vi "GeoData.vi"() -> ()   [LabVIEW 2017] (continued)
FL\tOrange County\tH1\n32733\t12095\tGoldenrod\tFL\tOrange County\tH1\n32792\t12095\tWinter park\tFL\tOrange County\tH1\n32768\t12095\tPlymouth\tFL\tOrange County\tH1\n32794\t12095\tMaitland\tFL\tOrange County\tH1\n32704\t12095\tApopka\tFL\tOrange County\tH1\n32709\t12095\tChristmas\tFL\tOrange County\tH1\n32818\t12095\tOrlando\tFL\tOrange County\tH1\n32803\t12095\tOrlando\tFL\tOrange County\tH1\n32806\t12095\tOrlando\tFL\tOrange County\tH1\n34761\t12095\tOcoee\tFL\tOrange County\tH1\n34786\t12095\tWindermere\tFL\tOrange County\tH1\n32856\t12095\tOrlando\tFL\tOrange County\tH1\n32703\t12095\tApopka\tFL\tOrange County\tH1\n32814\t12095\tOrlando\tFL\tOrange County\tH1\n32805\t12095\tOrlando\tFL\tOrange County\tH1\n32821\t12095\tOrlando\tFL\tOrange County\tH1\n32822\t12095\tOrlando\tFL\tOrange County\tH1\n32826\t12095\tOrlando\tFL\tOrange County\tH1\n32837\t12095\tOrlando\tFL\tOrange County\tH1\n32868\t12095\tOrlando\tFL\tOrange County\tH1\n32872\t12095\tOrlando\tFL\tOrange County\tH1\n32751\t12095\tMaitland\tFL\tOrange County\tH1\n32757\t12095\tMount dora\tFL\tOrange County\tH1\n34734\t12095\tGotha\tFL\tOrange County\tH1\n32860\t12095\tOrlando\tFL\tOrange County\tH1\n32802\t12095\tOrlando\tFL\tOrange County\tH1\n34778\t12095\tWinter garden\tFL\tOrange County\tH1\n32790\t12095\tWinter park\tFL\tOrange County\tH1\n34740\t12095\tKillarney\tFL\tOrange County\tH1\n32834\t12095\tOrlando\tFL\tOrange County\tH1\n32812\t12095\tOrlando\tFL\tOrange County\tH1\n32825\t12095\tOrlando\tFL\tOrange County\tH1\n32819\t12095\tOrlando\tFL\tOrange County\tH1\n32810\t12095\tOrlando\tFL\tOrange County\tH1\n32869\t12095\tOrlando\tFL\tOrange County\tH1\n32829\t12095\tOrlando\tFL\tOrange County\tH1\n32857\t12095\tOrlando\tFL\tOrange County\tH1\n32862\t12095\tOrlando\tFL\tOrange County\tH1\n32808\t12095\tOrlando\tFL\tOrange County\tH1\n32809\t12095\tOrlando\tFL\tOrange County\tH1\n32811\t12095\tOrlando\tFL\tOrange County\tH1\n32827\t12095\tOrlando\tFL\tOrange County\tH1\n32807\t12095\tOrlando\tFL\tOrange County\tH1\n32801\t12095\tOrlando\tFL\tOrange County\tH1\n32839\t12095\tOrlando\tFL\tOrange County\tH1\n32853\t12095\tOrlando\tFL\tOrange County\tH1\n32833\t12095\tOrlando\tFL\tOrange County\tH1\n34787\t12095\tWinter garden\tFL\tOrange County\tH1\n32855\t12095\tOrlando\tFL\tOrange County\tH1\n32816\t12095\tOrlando\tFL\tOrange County\tH1\n32878\t12095\tOrlando\tFL\tOrange County\tH1\n32712\t12095\tApopka\tFL\tOrange County\tH1\n32836\t12095\tOrlando\tFL\tOrange County\tH1\n32820\t12095\tOrlando\tFL\tOrange County\tH1\n32789\t12095\tWinter park\tFL\tOrange County\tH1\n32859\t12095\tOrlando\tFL\tOrange County\tH1\n32854\t12095\tOrlando\tFL\tOrange County\tH1\n32831\t12095\tOrlando\tFL\tOrange County\tH1\n34746\t12097\tKissimmee\tFL\tOsceola County\tH1\n34747\t12097\tKissimmee\tFL\tOsceola County\tH1\n34742\t12097\tKissimmee\tFL\tOsceola County\tH1\n34745\t12097\tKissimmee\tFL\tOsceola County\tH1\n32830\t12097\tOrlando\tFL\tOsceola County\tH1\n34972\t12097\tOkeechobee\tFL\tOsceola County\tH1\n34741\t12097\tKissimmee\tFL\tOsceola County\tH1\n34769\t12097\tSaint cloud\tFL\tOsceola County\tH1\n34771\t12097\tSaint cloud\tFL\tOsceola County\tH1\n34744\t12097\tKissimmee\tFL\tOsceola County\tH1\n33848\t12097\tIntercession city\tFL\tOsceola County\tH1\n32821\t12097\tOrlando\tFL\tOsceola County\tH1\n32837\t12097\tOrlando\tFL\tOsceola County\tH1\n34714\t12097\tClermont\tFL\tOsceola County\tH1\n33897\t12097\tDavenport\tFL\tOsceola County\tH1\n34739\t12097\tKenansville\tFL\tOsceola County\tH1\n34773\t12097\tSaint cloud\tFL\tOsceola County\tH1\n34743\t12097\tKissimmee\tFL\tOsceola County\tH1\n34759\t12097\tKissimmee\tFL\tOsceola County\tH1\n34758\t12097\tKissimmee\tFL\tOsceola County\tH1\n34772\t12097\tSaint cloud\tFL\tOsceola County\tH1\n34770\t12097\tSaint cloud\tFL\tOsceola County\tH1\n33896\t12097\tDavenport\tFL\tOsceola County\tH1\n33403\t12099\tWest palm beach\tFL\tPalm Beach County\tH1\n33409\t12099\tWest palm beach\tFL\tPalm Beach County\tH1\n33412\t12099\tWest palm beach\tFL\tPalm Beach County\tH1\n33415\t12099\tWest palm beach\tFL\tPalm Beach County\tH1\n33417\t12099\tWest palm beach\tFL\tPalm Beach County\tH1\n33446\t12099\tDelray beach\tFL\tPalm Beach County\tH1\n33460\t12099\tLake worth\tFL\tPalm Beach County\tH1\n33434\t12099\tBoca raton\tFL\tPalm Beach County\tH1\n33436\t12099\tBoynton beach\tFL\tPalm Beach County\tH1\n33478\t12099\tJupiter\tFL\tPalm Beach County\tH1\n33476\t12099\tPahokee\tFL\tPalm Beach County\tH1\n33484\t12099\tDelray beach\tFL\tPalm Beach County\tH1\n33488\t12099\tBoca raton\tFL\tPalm Beach County\tH1\n33448\t12099\tDelray beach\tFL\tPalm Beach County\tH1\n33401\t12099\tWest palm beach\tFL\tPalm Beach County\tH1\n33411\t12099\tWest palm beach\tFL\tPalm Beach County\tH1\n33425\t12099\tBoynton beach\tFL\tPalm Beach County\tH1\n33435\t12099\tBoynton beach\tFL\tPalm Beach County\tH1\n33444\t12099\tDelray beach\tFL\tPalm Beach County\tH1\n33449\t12099\tLake worth\tFL\tPalm Beach County\tH1\n33487\t12099\tBoca raton\tFL\tPalm Beach County\tH1\n33464\t12099\tBoca raton\tFL\tPalm Beach County\tH1\n33413\t12099\tWest palm beach\tFL\tPalm Beach County\tH1\n33429\t12099\tBoca raton\tFL\tPalm Beach County\tH1\n33472\t12099\tBoynton beach\tFL\tPalm Beach County\tH1\n33498\t12099\tBoca raton\tFL\tPalm Beach County\tH1\n33497\t12099\tBoca raton\tFL\tPalm Beach County\tH1\n33410\t12099\tPalm beach gardens\tFL\tPalm Beach County\tH1\n33427\t12099\tBoca raton\tFL\tPalm Beach County\tH1\n33445\t12099\tDelray beach\tFL\tPalm Beach County\tH1\n33463\t12099\tLake worth\tFL\tPalm Beach County\tH1\n33473\t12099\tBoynton beach\tFL\tPalm Beach County\tH1\n33480\t12099\tPalm beach\tFL\tPalm Beach County\tH1\n33465\t12099\tLake worth\tFL\tPalm Beach County\tH1\n33499\t12099\tBoca raton\tFL\tPalm Beach County\tH1\n33405\t12099\tWest palm beach\tFL\tPalm Beach County\tH1\n33414\t12099\tWellington\tFL\tPalm Beach County\tH1\n33431\t12099\tBoca raton\tFL\tPalm Beach County\tH1\n33462\t12099\tLake worth\tFL\tPalm Beach County\tH1\n33467\t12099\tLake worth\tFL\tPalm Beach County\tH1\n33438\t12099\tCanal point\tFL\tPalm Beach County\tH1\n33486\t12099\tBoca raton\tFL\tPalm Beach County\tH1\n33493\t12099\tSouth bay\tFL\tPalm Beach County\tH1\n33468\t12099\tJupiter\tFL\tPalm Beach County\tH1\n33418\t12099\tPalm beach gardens\tFL\tPalm Beach County\tH1\n33430\t12099\tBelle glade\tFL\tPalm Beach County\tH1\n33440\t12099\tClewiston\tFL\tPalm Beach County\tH1\n33458\t12099\tJupiter\tFL\tPalm Beach County\tH1\n33461\t12099\tLake worth\tFL\tPalm Beach County\tH1\n33433\t12099\tBoca raton\tFL\tPalm Beach County\tH1\n33477\t12099\tJupiter\tFL\tPalm Beach County\tH1\n33496\t12099\tBoca raton\tFL\tPalm Beach County\tH1\n33466\t12099\tLake worth\tFL\tPalm Beach County\tH1\n33454\t12099\tGreenacres\tFL\tPalm Beach County\tH1\n33407\t12099\tWest palm beach\tFL\tPalm Beach County\tH1\n33421\t12099\tRoyal palm beach\tFL\tPalm Beach County\tH1\n33406\t12099\tWest palm beach\tFL\tPalm Beach County\tH1\n33419\t12099\tWest palm beach\tFL\tPalm Beach County\tH1\n33437\t12099\tBoynton beach\tFL\tPalm Beach County\tH1\n33482\t12099\tDelray beach\tFL\tPalm Beach County\tH1\n33404\t12099\tWest palm beach\tFL\tPalm Beach County\tH1\n33408\t12099\tNorth palm beach\tFL\tPalm Beach County\tH1\n33428\t12099\tBoca raton\tFL\tPalm Beach County\tH1\n33426\t12099\tBoynton beach\tFL\tPalm Beach County\tH1\n33402\t12099\tWest palm beach\tFL\tPalm Beach County\tH1\n33416\t12099\tWest palm beach\tFL\tPalm Beach County\tH1\n33424\t12099\tBoynton beach\tFL\tPalm Beach County\tH1\n33432\t12099\tBoca raton\tFL\tPalm Beach County\tH1\n33469\t12099\tJupiter\tFL\tPalm Beach County\tH1\n33470\t12099\tLoxahatchee\tFL\tPalm Beach County\tH1\n33483\t12099\tDelray beach\tFL\tPalm Beach County\tH1\n33481\t12099\tBoca raton\tFL\tPalm Beach County\tH1\n33422\t12099\tWest palm beach\tFL\tPalm Beach County\tH1\n33474\t12099\tBoynton beach\tFL\tPalm Beach County\tH1\n33420\t12099\tWest palm beach\tFL\tPalm Beach County\tH1\n33459\t12099\tLake harbor\tFL\tPalm Beach County\tH1\n34653\t12101\tNew port richey\tFL\tPasco County\tH1\n34667\t12101\tHudson\tFL\tPasco County\tH1\n34637\t12101\tLand o lakes\tFL\tPasco County\tH1\n34690\t12101\tHoliday\tFL\tPasco County\tH1\n33523\t12101\tDade city\tFL\tPasco County\tH1\n33597\t12101\tWebster\tFL\tPasco County\tH1\n33544\t12101\tWesley chapel\tFL\tPasco County\tH1\n33548\t12101\tLutz\tFL\tPasco County\tH1\n33524\t12101\tCrystal springs\tFL\tPasco County\tH1\n33593\t12101\tTrilby\tFL\tPasco County\tH1\n33537\t12101\tLacoochee\tFL\tPasco County\tH1\n33558\t12101\tLutz\tFL\tPasco County\tH1\n33525\t12101\tDade city\tFL\tPasco County\tH1\n34610\t12101\tSpring hill\tFL\tPasco County\tH1\n34689\t12101\tTarpon springs\tFL\tPasco County\tH1\n34656\t12101\tNew port richey\tFL\tPasco County\tH1\n33849\t12101\tKathleen\tFL\tPasco County\tH1\n34679\t12101\tAripeka\tFL\tPasco County\tH1\n33545\t12101\tWesley chapel\tFL\tPasco County\tH1\n33539\t12101\tZephyrhills\tFL\tPasco County\tH1\n33526\t12101\tDade city\tFL\tPasco County\tH1\n34692\t12101\tHoliday\tFL\tPasco County\tH1\n33549\t12101\tLutz\tFL\tPasco County\tH1\n33576\t12101\tSan antonio\tFL\tPasco County\tH1\n34652\t12101\tNew port richey\tFL\tPasco County\tH1\n34668\t12101\tPort richey\tFL\tPasco County\tH1\n34674\t12101\tHudson\tFL\tPasco County\tH1\n34673\t12101\tPort richey\tFL\tPasco County\tH1\n33559\t12101\tLutz\tFL\tPasco County\tH1\n33543\t12101\tWesley chapel\tFL\tPasco County\tH1\n33542\t12101\tZephyrhills\tFL\tPasco County\tH1\n34604\t12101\tBrooksville\tFL\tPasco County\tH1\n34654\t12101\tNew port richey\tFL\tPasco County\tH1\n34655\t12101\tNew port richey\tFL\tPasco County\tH1\n34639\t12101\tLand o lakes\tFL\tPasco County\tH1\n34691\t12101\tHoliday\tFL\tPasco County\tH1\n33541\t12101\tZephyrhills\tFL\tPasco County\tH1\n33540\t12101\tZephyrhills\tFL\tPasco County\tH1\n33556\t12101\tOdessa\tFL\tPasco County\tH1\n34638\t12101\tLand o lakes\tFL\tPasco County\tH1\n34669\t12101\tHudson\tFL\tPasco County\tH1\n33809\t12101\tLakeland\tFL\tPasco County\tH1\n34680\t12101\tElfers\tFL\tPasco County\tH1\n33574\t12101\tSaint leo\tFL\tPasco County\tH1\n33701\t12103\tSaint petersburg\tFL\tPinellas County\tH1\n33709\t12103\tSaint petersburg\tFL\tPinellas County\tH1\n33776\t12103\tSeminole\tFL\tPinellas County\tH1\n33763\t12103\tClearwater\tFL\tPinellas County\tH1\n33710\t12103\tSaint petersburg\tFL\tPinellas County\tH1\n33782\t12103\tPinellas park\tFL\tPinellas County\tH1\n33773\t12103\tLargo\tFL\tPinellas County\tH1\n33786\t12103\tBelleair beach\tFL\tPinellas County\tH1\n33734\t12103\tSaint petersburg\tFL\tPinellas County\tH1\n33705\t12103\tSaint petersburg\tFL\tPinellas County\tH1\n33772\t12103\tSeminole\tFL\tPinellas County\tH1\n33713\t12103\tSaint petersburg\tFL\tPinellas County\tH1\n34683\t12103\tPalm harbor\tFL\tPinellas County\tH1\n33742\t12103\tSaint petersburg\tFL\tPinellas County\tH1\n33743\t12103\tSaint petersburg\tFL\tPinellas County\tH1\n33775\t12103\tSeminole\tFL\tPinellas County\tH1\n34682\t12103\tPalm harbor\tFL\tPinellas County\tH1\n33707\t12103\tSaint petersburg\tFL\tPinellas County\tH1\n33733\t12103\tSaint petersburg\tFL\tPinellas County\tH1\n33766\t12103\tClearwater\tFL\tPinellas County\tH1\n33712\t12103\tSaint petersburg\tFL\tPinellas County\tH1\n33747\t12103\tSaint petersburg\tFL\tPinellas County\tH1\n34689\t12103\tTarpon springs\tFL\tPinellas County\tH1\n34697\t12103\tDunedin\tFL\tPinellas County\tH1\n33760\t12103\tClearwater\tFL\tPinellas County\tH1\n34698\t12103\tDunedin\tFL\tPinellas County\tH1\n33738\t12103\tSaint petersburg\tFL\tPinellas County\tH1\n33741\t12103\tSaint petersburg\tFL\tPinellas County\tH1\n33729\t12103\tSaint petersburg\tFL\tPinellas County\tH1\n33730\t12103\tSaint petersburg\tFL\tPinellas County\tH1\n33703\t12103\tSaint petersburg\tFL\tPinellas County\tH1\n33702\t12103\tSaint petersburg\tFL\tPinellas County\tH1\n33715\t12103\tSaint petersburg\tFL\tPinellas County\tH1\n33716\t12103\tSaint petersburg\tFL\tPinellas County\tH1\n33767\t12103\tClearwater beach\tFL\tPinellas County\tH1\n33778\t12103\tLargo\tFL\tPinellas County\tH1\n33781\t12103\tPinellas park\tFL\tPinellas County\tH1\n33744\t12103\tBay pines\tFL\tPinellas County\tH1\n34681\t12103\tCrystal beach\tFL\tPinellas County\tH1\n33626\t12103\tTampa\tFL\tPinellas County\tH1\n33706\t12103\tSaint petersburg\tFL\tPinellas County\tH1\n33755\t12103\tClearwater\tFL\tPinellas County\tH1\n33761\t12103\tClearwater\tFL\tPinellas County\tH1\n33771\t12103\tLargo\tFL\tPinellas County\tH1\n33736\t12103\tSaint petersburg\tFL\tPinellas County\tH1\n33765\t12103\tClearwater\tFL\tPinellas County\tH1\n33756\t12103\tClearwater\tFL\tPinellas County\tH1\n33774\t12103\tLargo\tFL\tPinellas County\tH1\n33785\t12103\tIndian rocks beach\tFL\tPinellas County\tH1\n34677\t12103\tOldsmar\tFL\tPinellas County\tH1\n34685\t12103\tPalm harbor\tFL\tPinellas County\tH1\n34688\t12103\tTarpon springs\tFL\tPinellas County\tH1\n33779\t12103\tLargo\tFL\tPinellas County\tH1\n34660\t12103\tOzona\tFL\tPinellas County\tH1\n33708\t12103\tSaint petersburg\tFL\tPinellas County\tH1\n33757\t12103\tClearwater\tFL\tPinellas County\tH1\n33764\t12103\tClearwater\tFL\tPinellas County\tH1\n33770\t12103\tLargo\tFL\tPinellas County\tH1\n33780\t12103\tPinellas park\tFL\tPinellas County\tH1\n34684\t12103\tPalm harbor\tFL\tPinellas County\tH1\n33758\t12103\tClearwater\tFL\tPinellas County\tH1\n33704\t12103\tSaint petersburg\tFL\tPinellas County\tH1\n33759\t12103\tClearwater\tFL\tPinellas County\tH1\n33711\t12103\tSaint petersburg\tFL\tPinellas County\tH1\n33714\t12103\tSaint petersburg\tFL\tPinellas County\tH1\n33762\t12103\tClearwater\tFL\tPinellas County\tH1\n33777\t12103\tSeminole\tFL\tPinellas County\tH1\n33731\t12103\tSaint petersburg\tFL\tPinellas County\tH1\n34695\t12103\tSafety harbor\tFL\tPinellas County\tH1\n33732\t12103\tSaint petersburg\tFL\tPinellas County\tH1\n33784\t12103\tSaint petersburg\tFL\tPinellas County\tH1\n33547\t12105\tLithia\tFL\tPolk County\tH1\n33843\t12105\tFrostproof\tFL\tPolk County\tH1\n33838\t12105\tDundee\tFL\tPolk County\tH1\n33835\t12105\tBradley\tFL\tPolk County\tH1\n33855\t12105\tIndian lake estates\tFL\tPolk County\tH1\n33844\t12105\tHaines city\tFL\tPolk County\tH1\n33825\t12105\tAvon park\tFL\tPolk County\tH1\n33868\t12105\tPolk city\tFL\tPolk County\tH1\n33804\t12105\tLakeland\tFL\tPolk County\tH1\n33846\t12105\tHighland city\tFL\tPolk County\tH1\n33847\t12105\tHomeland\tFL\tPolk County\tH1\n33854\t12105\tLakeshore\tFL\tPolk County\tH1\n33801\t12105\tLakeland\tFL\tPolk County\tH1\n33837\t12105\tDavenport\tFL\tPolk County\tH1\n33813\t12105\tLakeland\tFL\tPolk County\tH1\n33823\t12105\tAuburndale\tFL\tPolk County\tH1\n33827\t12105\tBabson park\tFL\tPolk County\tH1\n33853\t12105\tLake wales\tFL\tPolk County\tH1\n33841\t12105\tFort meade\tFL\tPolk County\tH1\n33836\t12105\tDavenport\tFL\tPolk County\tH1\n33849\t12105\tKathleen\tFL\tPolk County\tH1\n33820\t12105\tAlturas\tFL\tPolk County\tH1\n33856\t12105\tNalcrest\tFL\tPolk County\tH1\n33863\t12105\tNichols\tFL\tPolk County\tH1\n33805\t12105\tLakeland\tFL\tPolk County\tH1\n33802\t12105\tLakeland\tFL\tPolk County\tH1\n33831\t12105\tBartow\tFL\tPolk County\tH1\n33851\t12105\tLake hamilton\tFL\tPolk County\tH1\n34714\t12105\tClermont\tFL\tPolk County\tH1\n33830\t12105\tBartow\tFL\tPolk County\tH1\n33897\t12105\tDavenport\tFL\tPolk County\tH1\n33812\t12105\tLakeland\tFL\tPolk County\tH1\n33834\t12105\tBowling green\tFL\tPolk County\tH1\n33839\t12105\tEagle lake\tFL\tPolk County\tH1\n33885\t12105\tWinter haven\tFL\tPolk County\tH1\n33840\t12105\tEaton park\tFL\tPolk County\tH1\n33845\t12105\tHaines city\tFL\tPolk County\tH1\n33867\t12105\tRiver ranch\tFL\tPolk County\tH1\n33860\t12105\tMulberry\tFL\tPolk County\tH1\n33810\t12105\tLakeland\tFL\tPolk County\tH1\n33881\t12105\tWinter haven\tFL\tPolk County\tH1\n33898\t12105\tLake wales\tFL\tPolk County\tH1\n33806\t12105\tLakeland\tFL\tPolk County\tH1\n33803\t12105\tLakeland\tFL\tPolk County\tH1\n34759\t12105\tKissimmee\tFL\tPolk County\tH1\n33815\t12105\tLakeland\tFL\tPolk County\tH1\n33850\t12105\tLake alfred\tFL\tPolk County\tH1\n33807\t12105\tLakeland\tFL\tPolk County\tH1\n34758\t12105\tKissimmee\tFL\tPolk County\tH1\n33809\t12105\tLakeland\tFL\tPolk County\tH1\n33811\t12105\tLakeland\tFL\tPolk County\tH1\n33859\t12105\tLake wales\tFL\tPolk County\tH1\n33880\t12105\tWinter haven\tFL\tPolk County\tH1\n33884\t12105\tWinter haven\tFL\tPolk County\tH1\n33896\t12105\tDavenport\tFL\tPolk County\tH1\n33882\t12105\tWinter haven\tFL\tPolk County\tH1\n33883\t12105\tWinter haven\tFL\tPolk County\tH1\n33858\t12105\tLoughman\tFL\tPolk County\tH1\n33877\t12105\tWaverly\tFL\tPolk County\tH1\n32131\t12107\tEast palatka\tFL\tPutnam County\tH1\n32139\t12107\tGeorgetown\tFL\tPutnam County\tH1\n32147\t12107\tHollister\tFL\tPutnam County\tH1\n32007\t12107\tBostwick\tFL\tPutnam County\tH1\n32640\t12107\tHawthorne\tFL\tPutnam County\tH1\n32145\t12107\tHastings\tFL\tPutnam County\tH1\n32193\t12107\tWelaka\tFL\tPutnam County\tH1\n32134\t12107\tFort mc coy\tFL\tPutnam County\tH1\n32187\t12107\tSan mateo\tFL\tPutnam County\tH1\n32181\t12107\tPomona park\tFL\tPutnam County\tH1\n32656\t12107\tKeystone heights\tFL\tPutnam County\tH1\n32189\t12107\tSatsuma\tFL\tPutnam County\tH1\n32148\t12107\tInterlachen\tFL\tPutnam County\tH1\n32140\t12107\tFlorahome\tFL\tPutnam County\tH1\n32185\t12107\tPutnam hall\tFL\tPutnam County\tH1\n32043\t12107\tGreen cove springs\tFL\tPutnam County\tH1\n32666\t12107\tMelrose\tFL\tPutnam County\tH1\n32138\t12107\tGrandin\tFL\tPutnam County\tH1\n32177\t12107\tPalatka\tFL\tPutnam County\tH1\n32112\t12107\tCrescent city\tFL\tPutnam County\tH1\n32131\t12109\tEast palatka\tFL\tSt. Johns County\tH1\n32085\t12109\tSaint augustine\tFL\tSt. Johns County\tH1\n32250\t12109\tJacksonville beach\tFL\tSt. Johns County\tH1\n32145\t12109\tHastings\tFL\tSt. Johns County\tH1\n32082\t12109\tPonte vedra beach\tFL\tSt. Johns County\tH1\n32081\t12109\tPonte vedra\tFL\tSt. Johns County\tH1\n32224\t12109\tJacksonville\tFL\tSt. Johns County\tH1\n32033\t12109\tElkton\tFL\tSt. Johns County\tH1\n32084\t12109\tSaint augustine\tFL\tSt. Johns County\tH1\n32092\t12109\tSaint augustine\tFL\tSt. Johns County\tH1\n32086\t12109\tSaint augustine\tFL\tSt. Johns County\tH1\n32095\t12109\tSaint augustine\tFL\tSt. Johns County\tH1\n32260\t12109\tJacksonville\tFL\tSt. Johns County\tH1\n32259\t12109\tSaint johns\tFL\tSt. Johns County\tH1\n32004\t12109\tPonte vedra beach\tFL\tSt. Johns County\tH1\n32080\t12109\tSaint augustine\tFL\tSt. Johns County\tH1\n34951\t12111\tFort pierce\tFL\tSt. Lucie County\tH1\n34981\t12111\tFort pierce\tFL\tSt. Lucie County\tH1\n34972\t12111\tOkeechobee\tFL\tSt. Lucie County\tH1\n34949\t12111\tFort pierce\tFL\tSt. Lucie County\tH1\n34974\t12111\tOkeechobee\tFL\tSt. Lucie County\tH1\n34957\t12111\tJensen beach\tFL\tSt. Lucie County\tH1\n34986\t12111\tPort saint lucie\tFL\tSt. Lucie County\tH1\n34979\t12111\tFort pierce\tFL\tSt. Lucie County\tH1\n34950\t12111\tFort pierce\tFL\tSt. Lucie County\tH1\n34952\t12111\tPort saint lucie\tFL\tSt. Lucie County\tH1\n34984\t12111\tPort saint lucie\tFL\tSt. Lucie County\tH1\n34946\t12111\tFort pierce\tFL\tSt. Lucie County\tH1\n34987\t12111\tPort saint lucie\tFL\tSt. Lucie County\tH1\n34983\t12111\tPort saint lucie\tFL\tSt. Lucie County\tH1\n34947\t12111\tFort pierce\tFL\tSt. Lucie County\tH1\n34985\t12111\tPort saint lucie\tFL\tSt. Lucie County\tH1\n34953\t12111\tPort saint lucie\tFL\tSt. Lucie County\tH1\n34990\t12111\tPalm city\tFL\tSt. Lucie County\tH1\n34945\t12111\tFort pierce\tFL\tSt. Lucie County\tH1\n34954\t12111\tFort pierce\tFL\tSt. Lucie County\tH1\n34982\t12111\tFort pierce\tFL\tSt. Lucie County\tH1\n34988\t12111\tPort saint lucie\tFL\tSt. Lucie County\tH1\n34948\t12111\tFort pierce\tFL\tSt. Lucie County\tH1\n32571\t12113\tMilton\tFL\tSanta Rosa County\tH1\n32562\t12113\tGulf breeze\tFL\tSanta Rosa County\tH1\n32570\t12113\tMilton\tFL\tSanta Rosa County\tH1\n32583\t12113\tMilton\tFL\tSanta Rosa County\tH1\n32572\t12113\tMilton\tFL\tSanta Rosa County\tH1\n32561\t12113\tGulf breeze\tFL\tSanta Rosa County\tH1\n32564\t12113\tHolt\tFL\tSanta Rosa County\tH1\n32530\t12113\tBagdad\tFL\tSanta Rosa County\tH1\n32566\t12113\tNavarre\tFL\tSanta Rosa County\tH1\n32569\t12113\tMary esther\tFL\tSanta Rosa County\tH1\n32531\t12113\tBaker\tFL\tSanta Rosa County\tH1\n32563\t12113\tGulf breeze\tFL\tSanta Rosa County\tH1\n32565\t12113\tJay\tFL\tSanta Rosa County\tH1\n34223\t12115\tEnglewood\tFL\tSarasota County\tH1\n34275\t12115\tNokomis\tFL\tSarasota County\tH1\n34290\t12115\tNorth port\tFL\tSarasota County\tH1\n34231\t12115\tSarasota\tFL\tSarasota County\tH1\n34237\t12115\tSarasota\tFL\tSarasota County\tH1\n34251\t12115\tMyakka city\tFL\tSarasota County\tH1\n34243\t12115\tSarasota\tFL\tSarasota County\tH1\n34287\t12115\tNorth port\tFL\tSarasota County\tH1\n34293\t12115\tVenice\tFL\tSarasota County\tH1\n34292\t12115\tVenice\tFL\tSarasota County\tH1\n34272\t12115\tLaurel\tFL\tSarasota County\tH1\n34228\t12115\tLongboat key\tFL\tSarasota County\tH1\n34232\t12115\tSarasota\tFL\tSarasota County\tH1\n34239\t12115\tSarasota\tFL\tSarasota County\tH1\n34224\t12115\tEnglewood\tFL\tSarasota County\tH1\n34229\t12115\tOsprey\tFL\tSarasota County\tH1\n34240\t12115\tSarasota\tFL\tSarasota County\tH1\n34285\t12115\tVenice\tFL\tSarasota County\tH1\n34266\t12115\tArcadia\tFL\tSarasota County\tH1\n34242\t12115\tSarasota\tFL\tSarasota County\tH1\n34291\t12115\tNorth port\tFL\tSarasota County\tH1\n34276\t12115\tSarasota\tFL\tSarasota County\tH1\n34277\t12115\tSarasota\tFL\tSarasota County\tH1\n34249\t12115\tSarasota\tFL\tSarasota County\tH1\n34238\t12115\tSarasota\tFL\tSarasota County\tH1\n34230\t12115\tSarasota\tFL\tSarasota County\tH1\n34288\t12115\tNorth port\tFL\tSarasota County\tH1\n34289\t12115\tNorth port\tFL\tSarasota County\tH1\n34284\t12115\tVenice\tFL\tSarasota County\tH1\n34295\t12115\tEnglewood\tFL\tSarasota County\tH1\n34235\t12115\tSarasota\tFL\tSarasota County\tH1\n34241\t12115\tSarasota\tFL\tSarasota County\tH1\n34233\t12115\tSarasota\tFL\tSarasota County\tH1\n34234\t12115\tSarasota\tFL\tSarasota County\tH1\n34236\t12115\tSarasota\tFL\tSarasota County\tH1\n34286\t12115\tNorth port\tFL\tSarasota County\tH1\n34274\t12115\tNokomis\tFL\tSarasota County\tH1\n32701\t12117\tAltamonte springs\tFL\tSeminole County\tH1\n32708\t12117\tWinter springs\tFL\tSeminole County\tH1\n32714\t12117\tAltamonte springs\tFL\tSeminole County\tH1\n32773\t12117\tSanford\tFL\tSeminole County\tH1\n32779\t12117\tLongwood\tFL\tSeminole County\tH1\n32719\t12117\tWinter springs\tFL\tSeminole County\tH1\n32765\t12117\tOviedo\tFL\tSeminole County\tH1\n32716\t12117\tAltamonte springs\tFL\tSeminole County\tH1\n32752\t12117\tLongwood\tFL\tSeminole County\tH1\n32795\t12117\tLake mary\tFL\tSeminole County\tH1\n32707\t12117\tCasselberry\tFL\tSeminole County\tH1\n32792\t12117\tWinter park\tFL\tSeminole County\tH1\n32762\t12117\tOviedo\tFL\tSeminole County\tH1\n32772\t12117\tSanford\tFL\tSeminole County\tH1\n32746\t12117\tLake mary\tFL\tSeminole County\tH1\n32750\t12117\tLongwood\tFL\tSeminole County\tH1\n32771\t12117\tSanford\tFL\tSeminole County\tH1\n32730\t12117\tCasselberry\tFL\tSeminole County\tH1\n32718\t12117\tCasselberry\tFL\tSeminole County\tH1\n32703\t12117\tApopka\tFL\tSeminole County\tH1\n32715\t12117\tAltamonte springs\tFL\tSeminole County\tH1\n32751\t12117\tMaitland\tFL\tSeminole County\tH1\n32766\t12117\tOviedo\tFL\tSeminole County\tH1\n32791\t12117\tLongwood\tFL\tSeminole County\tH1\n32799\t12117\tMid florida\tFL\tSeminole County\tH1\n32732\t12117\tGeneva\tFL\tSeminole County\tH1\n32747\t12117\tLake monroe\tFL\tSeminole County\tH1\n34731\t12119\tFruitland park\tFL\tSumter County\tH1\n33597\t12119\tWebster\tFL\tSumter County\tH1\n34491\t12119\tSummerfield\tFL\tSumter County\tH1\n32163\t12119\tThe villages\tFL\tSumter County\tH1\n33513\t12119\tBushnell\tFL\tSumter County\tH1\n32159\t12119\tLady lake\tFL\tSumter County\tH1\n33514\t12119\tCenter hill\tFL\tSumter County\tH1\n33538\t12119\tLake panasoffkee\tFL\tSumter County\tH1\n34785\t12119\tWildwood\tFL\tSumter County\tH1\n33585\t12119\tSumterville\tFL\tSumter County\tH1\n34484\t12119\tOxford\tFL\tSumter County\tH1\n32162\t12119\tThe villages\tFL\tSumter County\tH1\n33521\t12119\tColeman\tFL\tSumter County\tH1\n32038\t12121\tFort white\tFL\tSuwannee County\tH1\n32008\t12121\tBranford\tFL\tSuwannee County\tH1\n32062\t12121\tMc alpin\tFL\tSuwannee County\tH1\n32060\t12121\tLive oak\tFL\tSuwannee County\tH1\n32071\t12121\tO brien\tFL\tSuwannee County\tH1\n32096\t12121\tWhite springs\tFL\tSuwannee County\tH1\n32064\t12121\tLive oak\tFL\tSuwannee County\tH1\n32024\t12121\tLake city\tFL\tSuwannee County\tH1\n32055\t12121\tLake city\tFL\tSuwannee County\tH1\n32094\t12121\tWellborn\tFL\tSuwannee County\tH1\n32357\t12123\tShady grove\tFL\tTaylor County\tH1\n32331\t12123\tGreenville\tFL\tTaylor County\tH1\n32356\t12123\tSalem\tFL\tTaylor County\tH1\n32336\t12123\tLamont\tFL\tTaylor County\tH1\n32348\t12123\tPerry\tFL\tTaylor County\tH1\n32359\t12123\tSteinhatchee\tFL\tTaylor County\tH1\n32347\t12123\tPerry\tFL\tTaylor County\tH1\n32058\t12125\tLawtey\tFL\tUnion County\tH1\n32697\t12125\tWorthington springs\tFL\tUnion County\tH1\n32083\t12125\tRaiford\tFL\tUnion County\tH1\n32054\t12125\tLake butler\tFL\tUnion County\tH1\n32170\t12127\tNew smyrna beach\tFL\tVolusia County\tH1\n32117\t12127\tDaytona beach\tFL\tVolusia County\tH1\n32119\t12127\tDaytona beach\tFL\tVolusia County\tH1\n32713\t12127\tDebary\tFL\tVolusia County\tH1\n32180\t12127\tPierson\tFL\tVolusia County\tH1\n32126\t12127\tDaytona beach\tFL\tVolusia County\tH1\n32759\t12127\tOak hill\tFL\tVolusia County\tH1\n32130\t12127\tDe leon springs\tFL\tVolusia County\tH1\n32121\t12127\tDaytona beach\tFL\tVolusia County\tH1\n32122\t12127\tDaytona beach\tFL\tVolusia County\tH1\n32127\t12127\tPort orange\tFL\tVolusia County\tH1\n32118\t12127\tDaytona beach\tFL\tVolusia County\tH1\n32724\t12127\tDeland\tFL\tVolusia County\tH1\n32114\t12127\tDaytona beach\tFL\tVolusia County\tH1\n32141\t12127\tEdgewater\tFL\tVolusia County\tH1\n32169\t12127\tNew smyrna beach\tFL\tVolusia County\tH1\n32128\t12127\tPort orange\tFL\tVolusia County\tH1\n32753\t12127\tDebary\tFL\tVolusia County\tH1\n32175\t12127\tOrmond beach\tFL\tVolusia County\tH1\n32723\t12127\tDeland\tFL\tVolusia County\tH1\n32706\t12127\tCassadaga\tFL\tVolusia County\tH1\n32124\t12127\tDaytona beach\tFL\tVolusia County\tH1\n32173\t12127\tOrmond beach\tFL\tVolusia County\tH1\n32105\t12127\tBarberville\tFL\tVolusia County\tH1\n32136\t12127\tFlagler beach\tFL\tVolusia County\tH1\n32764\t12127\tOsteen\tFL\tVolusia County\tH1\n32721\t12127\tDeland\tFL\tVolusia County\tH1\n32174\t12127\tOrmond beach\tFL\tVolusia County\tH1\n32176\t12127\tOrmond beach\tFL\tVolusia County\tH1\n32132\t12127\tEdgewater\tFL\tVolusia County\tH1\n32754\t12127\tMims\tFL\tVolusia County\tH1\n32115\t12127\tDaytona beach\tFL\tVolusia County\tH1\n32102\t12127\tAstor\tFL\tVolusia County\tH1\n32728\t12127\tDeltona\tFL\tVolusia County\tH1\n32168\t12127\tNew smyrna beach\tFL\tVolusia County\tH1\n32190\t12127\tSeville\tFL\tVolusia County\tH1\n32763\t12127\tOrange city\tFL\tVolusia County\tH1\n32738\t12127\tDeltona\tFL\tVolusia County\tH1\n32774\t12127\tOrange city\tFL\tVolusia County\tH1\n32120\t12127\tDaytona beach\tFL\tVolusia County\tH1\n32125\t12127\tDaytona beach\tFL\tVolusia County\tH1\n32198\t12127\tDaytona beach\tFL\tVolusia County\tH1\n32129\t12127\tPort orange\tFL\tVolusia County\tH1\n32720\t12127\tDeland\tFL\tVolusia County\tH1\n32725\t12127\tDeltona\tFL\tVolusia County\tH1\n32732\t12127\tGeneva\tFL\tVolusia County\tH1\n32744\t12127\tLake helen\tFL\tVolusia County\tH1\n32112\t12127\tCrescent city\tFL\tVolusia County\tH1\n32739\t12127\tDeltona\tFL\tVolusia County\tH1\n32326\t12129\tCrawfordville\tFL\tWakulla County\tH1\n32358\t12129\tSopchoppy\tFL\tWakulla County\tH1\n32327\t12129\tCrawfordville\tFL\tWakulla County\tH1\n32346\t12129\tPanacea\tFL\tWakulla County\tH1\n32355\t12129\tSaint marks\tFL\tWakulla County\tH1\n32455\t12131\tPonce de leon\tFL\tWalton County\tH1\n32539\t12131\tCrestview\tFL\tWalton County\tH1\n32578\t12131\tNiceville\tFL\tWalton County\tH1\n32459\t12131\tSanta rosa beach\tFL\tWalton County\tH1\n32538\t12131\tPaxton\tFL\tWalton County\tH1\n32461\t12131\tInlet beach\tFL\tWalton County\tH1\n32464\t12131\tWestville\tFL\tWalton County\tH1\n32462\t12131\tVernon\tFL\tWalton County\tH1\n32407\t12131\tPanama city beach\tFL\tWalton County\tH1\n32435\t12131\tDefuniak springs\tFL\tWalton County\tH1\n32433\t12131\tDefuniak springs\tFL\tWalton County\tH1\n32550\t12131\tMiramar beach\tFL\tWalton County\tH1\n32422\t12131\tArgyle\tFL\tWalton County\tH1\n32439\t12131\tFreeport\tFL\tWalton County\tH1\n32567\t12131\tLaurel hill\tFL\tWalton County\tH1\n32428\t12133\tChipley\tFL\tWashington County\tH1\n32420\t12133\tAlford\tFL\tWashington County\tH1\n32437\t12133\tEbro\tFL\tWashington County\tH1\n32438\t12133\tFountain\tFL\tWashington County\tH1\n32431\t12133\tCottondale\tFL\tWashington County\tH1\n32427\t12133\tCaryville\tFL\tWashington County\tH1\n32462\t12133\tVernon\tFL\tWashington County\tH1\n32425\t12133\tBonifay\tFL\tWashington County\tH1\n32466\t12133\tYoungstown\tFL\tWashington County\tH1\n32463\t12133\tWausau\tFL\tWashington County\tH1\n31557\t13001\tPatterson\tGA\tAppling County\tH1\n31513\t13001\tBaxley\tGA\tAppling County\tH1\n31518\t13001\tBristol\tGA\tAppling County\tH1\n31539\t13001\tHazlehurst\tGA\tAppling County\tH1\n31560\t13001\tScreven\tGA\tAppling County\tH1\n31563\t13001\tSurrency\tGA\tAppling County\tH1\n31555\t13001\tOdum\tGA\tAppling County\tH1\n30233\t13001\tJackson\tGA\tAppling County\tH1\n31510\t13001\tAlma\tGA\tAppling County\tH1\n31552\t13003\tMillwood\tGA\tAtkinson County\tH1\n31624\t13003\tAxson\tGA\tAtkinson County\tH1\n31642\t13003\tPearson\tGA\tAtkinson County\tH1\n31650\t13003\tWillacoochee\tGA\tAtkinson County\tH1\n31635\t13003\tLakeland\tGA\tAtkinson County\tH1\n31551\t13005\tMershon\tGA\tBacon County\tH1\n31513\t13005\tBaxley\tGA\tBacon County\tH1\n31518\t13005\tBristol\tGA\tBacon County\tH1\n31554\t13005\tNicholls\tGA\tBacon County\tH1\n31510\t13005\tAlma\tGA\tBacon County\tH1\n39841\t13007\tDamascus\tGA\tBaker County\tH1\n31721\t13007\tAlbany\tGA\tBaker County\tH1\n39862\t13007\tLeary\tGA\tBaker County\tH1\n39870\t13007\tNewton\tGA\tBaker County\tH1\n39813\t13007\tArlington\tGA\tBaker County\tH1\n39837\t13007\tColquitt\tGA\tBaker County\tH1\n31033\t13009\tHaddock\tGA\tBaldwin County\tH1\n31031\t13009\tGordon\tGA\tBaldwin County\tH1\n31059\t13009\tMilledgeville\tGA\tBaldwin County\tH1\n31062\t13009\tMilledgeville\tGA\tBaldwin County\tH1\n31034\t13009\tHardwick\tGA\tBaldwin County\tH1\n31061\t13009\tMilledgeville\tGA\tBaldwin County\tH1\n31082\t13009\tSandersville\tGA\tBaldwin County\tH1\n31087\t13009\tSparta\tGA\tBaldwin County\tH1\n30511\t13011\tBaldwin\tGA\tBanks County\tH1\n30510\t13011\tAlto\tGA\tBanks County\tH1\n30529\t13011\tCommerce\tGA\tBanks County\tH1\n30558\t13011\tMaysville\tGA\tBanks County\tH1\n30633\t13011\tDanielsville\tGA\tBanks County\tH1\n30543\t13011\tGillsville\tGA\tBanks County\tH1\n30521\t13011\tCarnesville\tGA\tBanks County\tH1\n30547\t13011\tHomer\tGA\tBanks County\tH1\n30577\t13011\tToccoa\tGA\tBanks County\tH1\n30530\t13011\tCommerce\tGA\tBanks County\tH1\n30554\t13011\tLula\tGA\tBanks County\tH1\n30548\t13013\tHoschton\tGA\tBarrow County\tH1\n30620\t13013\tBethlehem\tGA\tBarrow County\tH1\n30011\t13013\tAuburn\tGA\tBarrow County\tH1\n30622\t13013\tBogart\tGA\tBarrow County\tH1\n30656\t13013\tMonroe\tGA\tBarrow County\tH1\n30517\t13013\tBraselton\tGA\tBarrow County\tH1\n30680\t13013\tWinder\tGA\tBarrow County\tH1\n30666\t13013\tStatham\tGA\tBarrow County\tH1\n30123\t13015\tCassville\tGA\tBartow County\tH1\n30137\t13015\tEmerson\tGA\tBartow County\tH1\n30178\t13015\tTaylorsville\tGA\tBartow County\tH1\n30171\t13015\tRydal\tGA\tBartow County\tH1\n30102\t13015\tAcworth\tGA\tBartow County\tH1\n30103\t13015\tAdairsville\tGA\tBartow County\tH1\n30184\t13015\tWhite\tGA\tBartow County\tH1\n30101\t13015\tAcworth\tGA\tBartow County\tH1\n30104\t13015\tAragon\tGA\tBartow County\tH1\n30139\t13015\tFairmount\tGA\tBartow County\tH1\n30161\t13015\tRome\tGA\tBartow County\tH1\n30145\t13015\tKingston\tGA\tBartow County\tH1\n30183\t13015\tWaleska\tGA\tBartow County\tH1\n30120\t13015\tCartersville\tGA\tBartow County\tH1\n30121\t13015\tCartersville\tGA\tBartow County\tH1\n31001\t13017\tAbbeville\tGA\tBen Hill County\tH1\n31798\t13017\tWray\tGA\tBen Hill County\tH1\n31079\t13017\tRochelle\tGA\tBen Hill County\tH1\n31750\t13017\tFitzgerald\tGA\tBen Hill County\tH1\n31783\t13017\tRebecca\tGA\tBen Hill County\tH1\n31622\t13019\tAlapaha\tGA\tBerrien County\tH1\n31774\t13019\tOcilla\tGA\tBerrien County\tH1\n31637\t13019\tLenox\tGA\tBerrien County\tH1\n31645\t13019\tRay city\tGA\tBerrien County\tH1\n31635\t13019\tLakeland\tGA\tBerrien County\tH1\n31639\t13019\tNashville\tGA\tBerrien County\tH1\n31749\t13019\tEnigma\tGA\tBerrien County\tH1\n31794\t13019\tTifton\tGA\tBerrien County\tH1\n31211\t13021\tMacon\tGA\tBibb County\tH1\n31203\t13021\tMacon\tGA\tBibb County\tH1\n31213\t13021\tMacon\tGA\tBibb County\tH1\n31208\t13021\tMacon\tGA\tBibb County\tH1\n31201\t13021\tMacon\tGA\tBibb County\tH1\n31216\t13021\tMacon\tGA\tBibb County\tH1\n31220\t13021\tMacon\tGA\tBibb County\tH1\n31207\t13021\tMacon\tGA\tBibb County\tH1\n31206\t13021\tMacon\tGA\tBibb County\tH1\n31205\t13021\tMacon\tGA\tBibb County\tH1\n31209\t13021\tMacon\tGA\tBibb County\tH1\n31066\t13021\tMusella\tGA\tBibb County\tH1\n31204\t13021\tMacon\tGA\tBibb County\tH1\n31217\t13021\tMacon\tGA\tBibb County\tH1\n31020\t13021\tDry branch\tGA\tBibb County\tH1\n31052\t13021\tLizella\tGA\tBibb County\tH1\n31221\t13021\tMacon\tGA\tBibb County\tH1\n31295\t13021\tMacon\tGA\tBibb County\tH1\n31210\t13021\tMacon\tGA\tBibb County\tH1\n31036\t13023\tHawkinsville\tGA\tBleckley County\tH1\n31022\t13023\tDudley\tGA\tBleckley County\tH1\n31014\t13023\tCochran\tGA\tBleckley County\tH1\n31012\t13023\tChester\tGA\tBleckley County\tH1\n31017\t13023\tDanville\tGA\tBleckley County\tH1\n31065\t13023\tMontrose\tGA\tBleckley County\tH1\n31543\t13025\tHortense\tGA\tBrantley County\tH1\n31557\t13025\tPatterson\tGA\tBrantley County\tH1\n31542\t13025\tHoboken\tGA\tBrantley County\tH1\n31537\t13025\tFolkston\tGA\tBrantley County\tH1\n31565\t13025\tWaverly\tGA\tBrantley County\tH1\n31503\t13025\tWaycross\tGA\tBrantley County\tH1\n31566\t13025\tWaynesville\tGA\tBrantley County\tH1\n31553\t13025\tNahunta\tGA\tBrantley County\tH1\n31625\t13027\tBarney\tGA\tBrooks County\tH1\n31778\t13027\tPavo\tGA\tBrooks County\tH1\n31788\t13027\tMoultrie\tGA\tBrooks County\tH1\n31638\t13027\tMorven\tGA\tBrooks County\tH1\n31629\t13027\tDixie\tGA\tBrooks County\tH1\n31602\t13027\tValdosta\tGA\tBrooks County\tH1\n31643\t13027\tQuitman\tGA\tBrooks County\tH1\n31626\t13027\tBoston\tGA\tBrooks County\tH1\n31302\t13029\tBloomingdale\tGA\tBryan County\tH1\n31308\t13029\tEllabell\tGA\tBryan County\tH1\n31321\t13029\tPembroke\tGA\tBryan County\tH1\n31324\t13029\tRichmond hill\tGA\tBryan County\tH1\n31308\t13031\tEllabell\tGA\tBulloch County\tH1\n30460\t13031\tStatesboro\tGA\tBulloch County\tH1\n30450\t13031\tPortal\tGA\tBulloch County\tH1\n30452\t13031\tRegister\tGA\tBulloch County\tH1\n31321\t13031\tPembroke\tGA\tBulloch County\tH1\n30471\t13031\tTwin city\tGA\tBulloch County\tH1\n30417\t13031\tClaxton\tGA\tBulloch County\tH1\n30439\t13031\tMetter\tGA\tBulloch County\tH1\n30459\t13031\tStatesboro\tGA\tBulloch County\tH1\n30458\t13031\tStatesboro\tGA\tBulloch County\tH1\n30415\t13031\tBrooklet\tGA\tBulloch County\tH1\n30425\t13031\tGarfield\tGA\tBulloch County\tH1\n30461\t13031\tStatesboro\tGA\tBulloch County\tH1\n30426\t13033\tGirard\tGA\tBurke County\tH1\n30442\t13033\tMillen\tGA\tBurke County\tH1\n30815\t13033\tHephzibah\tGA\tBurke County\tH1\n30434\t13033\tLouisville\tGA\tBurke County\tH1\n30456\t13033\tSardis\tGA\tBurke County\tH1\n30805\t13033\tBlythe\tGA\tBurke County\tH1\n30830\t13033\tWaynesboro\tGA\tBurke County\tH1\n30441\t13033\tMidville\tGA\tBurke County\tH1\n30816\t13033\tKeysville\tGA\tBurke County\tH1\n30223\t13035\tGriffin\tGA\tButts County\tH1\n30234\t13035\tJenkinsburg\tGA\tButts County\tH1\n30224\t13035\tGriffin\tGA\tButts County\tH1\n31029\t13035\tForsyth\tGA\tButts County\tH1\n30216\t13035\tFlovilla\tGA\tButts County\tH1\n30248\t13035\tLocust grove\tGA\tButts County\tH1\n30233\t13035\tJackson\tGA\tButts County\tH1\n39840\t13037\tCuthbert\tGA\tCalhoun County\tH1\n39866\t13037\tMorgan\tGA\tCalhoun County\tH1\n39842\t13037\tDawson\tGA\tCalhoun County\tH1\n39846\t13037\tEdison\tGA\tCalhoun County\tH1\n39862\t13037\tLeary\tGA\tCalhoun County\tH1\n39886\t13037\tShellman\tGA\tCalhoun County\tH1\n39813\t13037\tArlington\tGA\tCalhoun County\tH1\n31548\t13039\tKingsland\tGA\tCamden County\tH1\n31568\t13039\tWhite oak\tGA\tCamden County\tH1\n31537\t13039\tFolkston\tGA\tCamden County\tH1\n31569\t13039\tWoodbine\tGA\tCamden County\tH1\n31565\t13039\tWaverly\tGA\tCamden County\tH1\n31558\t13039\tSaint marys\tGA\tCamden County\tH1\n31566\t13039\tWaynesville\tGA\tCamden County\tH1\n31547\t13039\tKings bay\tGA\tCamden County\tH1\n30420\t13043\tCobbtown\tGA\tCandler County\tH1\n30452\t13043\tRegister\tGA\tCandler County\tH1\n30471\t13043\tTwin city\tGA\tCandler County\tH1\n30439\t13043\tMetter\tGA\tCandler County\tH1\n30451\t13043\tPulaski\tGA\tCandler County\tH1\n30179\t13045\tTemple\tGA\tCarroll County\tH1\n30185\t13045\tWhitesburg\tGA\tCarroll County\tH1\n30108\t13045\tBowdon\tGA\tCarroll County\tH1\n30118\t13045\tCarrollton\tGA\tCarroll County\tH1\n30187\t13045\tWinston\tGA\tCarroll County\tH1\n30150\t13045\tMount zion\tGA\tCarroll County\tH1\n30112\t13045\tCarrollton\tGA\tCarroll County\tH1\n30180\t13045\tVilla rica\tGA\tCarroll County\tH1\n30109\t13045\tBowdon junction\tGA\tCarroll County\tH1\n30110\t13045\tBremen\tGA\tCarroll County\tH1\n30116\t13045\tCarrollton\tGA\tCarroll County\tH1\n30170\t13045\tRoopville\tGA\tCarroll County\tH1\n30119\t13045\tCarrollton\tGA\tCarroll County\tH1\n30117\t13045\tCarrollton\tGA\tCarroll County\tH1\n30182\t13045\tWaco\tGA\tCarroll County\tH1\n30707\t13047\tChickamauga\tGA\tCatoosa County\tH1\n30741\t13047\tRossville\tGA\tCatoosa County\tH1\n30736\t13047\tRinggold\tGA\tCatoosa County\tH1\n30710\t13047\tCohutta\tGA\tCatoosa County\tH1\n30742\t13047\tFort oglethorpe\tGA\tCatoosa County\tH1\n30755\t13047\tTunnel hill\tGA\tCatoosa County\tH1\n30739\t13047\tRock spring\tGA\tCatoosa County\tH1\n30726\t13047\tGraysville\tGA\tCatoosa County\tH1\n31537\t13049\tFolkston\tGA\tCharlton County\tH1\n31631\t13049\tFargo\tGA\tCharlton County\tH1\n31562\t13049\tSaint george\tGA\tCharlton County\tH1\n31553\t13049\tNahunta\tGA\tCharlton County\tH1\n31302\t13051\tBloomingdale\tGA\tChatham County\tH1\n31408\t13051\tSavannah\tGA\tChatham County\tH1\n31411\t13051\tSavannah\tGA\tChatham County\tH1\n31410\t13051\tSavannah\tGA\tChatham County\tH1\n31420\t13051\tSavannah\tGA\tChatham County\tH1\n31312\t13051\tGuyton\tGA\tChatham County\tH1\n31322\t13051\tPooler\tGA\tChatham County\tH1\n31328\t13051\tTybee island\tGA\tChatham County\tH1\n31415\t13051\tSavannah\tGA\tChatham County\tH1\n31414\t13051\tSavannah\tGA\tChatham County\tH1\n31403\t13051\tSavannah\tGA\tChatham County\tH1\n31401\t13051\tSavannah\tGA\tChatham County\tH1\n31404\t13051\tSavannah\tGA\tChatham County\tH1\n31407\t13051\tPort wentworth\tGA\tChatham County\tH1\n31405\t13051\tSavannah\tGA\tChatham County\tH1\n31416\t13051\tSavannah\tGA\tChatham County\tH1\n31409\t13051\tSavannah\tGA\tChatham County\tH1\n31418\t13051\tSavannah\tGA\tChatham County\tH1\n31402\t13051\tSavannah\tGA\tChatham County\tH1\n31406\t13051\tSavannah\tGA\tChatham County\tH1\n31419\t13051\tSavannah\tGA\tChatham County\tH1\n31421\t13051\tSavannah\tGA\tChatham County\tH1\n31412\t13051\tSavannah\tGA\tChatham County\tH1\n31905\t13053\tFort benning\tGA\tChattahoochee County\tH1\n31805\t13053\tCusseta\tGA\tChattahoochee County\tH1\n31995\t13053\tFort benning\tGA\tChattahoochee County\tH1\n30105\t13055\tArmuchee
